vi "State_ExecCMD.vi"(6 "Callback":T1, 8 "error in (no error)":errorcluster, 9 "Parameter":variant, 10 "Command":string, 11 "MB Slave Simulator Base in":refnum<class "MB Slave Simulator Base.lvclass">) -> (0 "error out":errorcluster, 1 "Suppress Debug?":bool, 2 "Debug Message":string, 3 "MB Slave Simulator Base out":refnum<class "MB Slave Simulator Base.lvclass">)   [LabVIEW 2021, in "MB Slave Simulator Base.lvclass"]
uses:
  MB Slave Simulator Base.lvclass
  C:/Program Files (x86)/National Instruments/LabVIEW 2021/user.lib/S2 Labs/Module Framework/Modules/Modbus/Modbus Slave Base/Modbus Slave Base.lvclass
  <userlib>/S2 Labs/Module Framework/Modules/Base/Callback Typdef.ctl
  <userlib>/S2 Labs/Queued State Machine/Callback Notifier/Callback Notifier.lvclass
  <userlib>/S2 Labs/Queued State Machine/TypeDefs/CallbackNotifierRef.ctl
  TypeDefs/set_register_cmd_type.ctl
  <userlib>/S2 Labs/Module Framework/Modules/Modbus/Modbus Slave Base/Modbus Slave Base.lvclass/Modbus Slave Base.ctl
  <userlib>/S2 Labs/Queued State Machine/Callback Notifier/Callback Notifier.lvclass/Callback Notifier.ctl
  064588b5-2067-4a9b-8024-f71601e02561.vi
  780a900f-1216-485f-86c7-dbb916bac525.vi
  e8940690-14e9-4793-917b-da751b7dd203.vi
  <userlib>/S2 Labs/Module Framework/Modules/Modbus/Modbus Slave Base/Read MB Ref.vi
  <userlib>/S2 Labs/Queued State Machine/Callback Notifier/Read Callback Notifier Ref.vi
  <vilib>/Utility/error.llb/Error Cluster From Error Code.vi
  <vilib>/JDP Science/JSONtext/Variant to JSON Text.vi
  <userlib>/S2 Labs/Modbus Toolkit/Slave/S2L Modbus Slave.lvclass
  <vilib>/JDP Science/JSONtext/LVClass Serializer/JSONtext LVClass Serializer.lvclass
  <userlib>/S2 Labs/Module Framework/Modules/Modbus/Modbus Slave Base/Modbus Slave Base.lvclass
  <userlib>/S2 Labs/Queued State Machine/QSM.lvclass
  <userlib>/S2 Labs/Module Framework/Modules/Base/Module.lvclass
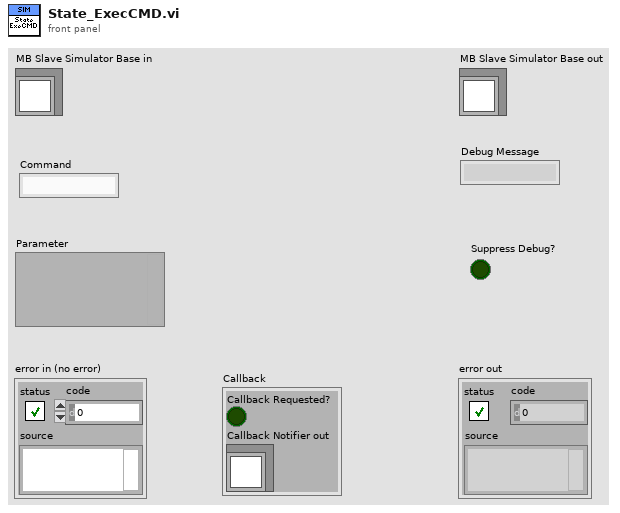
[diagram p1: front panel]
types:
  T1 = typedef "Module.lvclass/Callback Typdef.ctl" = cluster{"Callback Requested?":bool, "Callback Notifier out":T2}
  T2 = typedef "QSM.lvclass/CallbackNotifierRef.ctl" = refnum<class "Callback Notifier.lvclass">
  T3 = typedef "MB Slave Simulator Base.lvclass/set_register_cmd_type.ctl" = cluster{"Label":string, "Value":dbl}
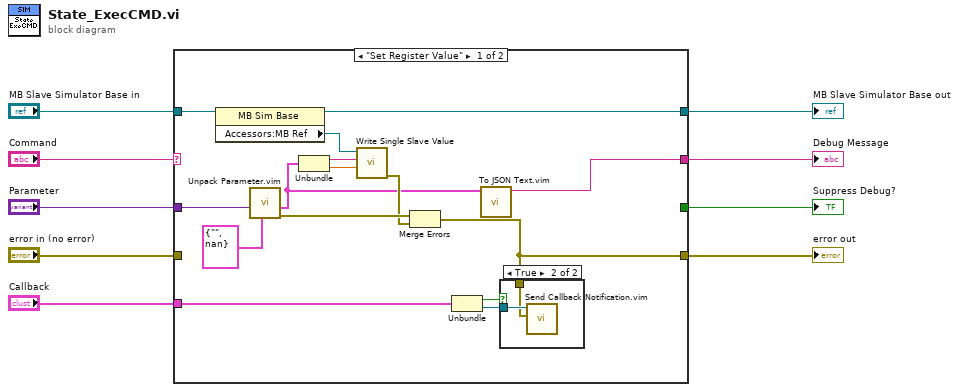
[diagram p0: block diagram]
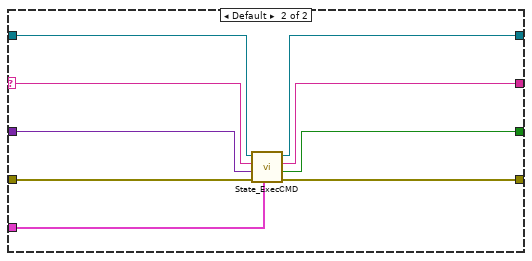
[diagram p3: hidden frame]
diagram:
  n1 = case shown="\"Set Register Value\"" "Command" {
    selector: "Command" -> [_ w28]
    tunnel: [w12 w35] -> w9
    tunnel: [_ w34] -> w8
    tunnel: [w10 w33] -> w7
    tunnel: [w23 w32] -> w6
    tunnel: "Callback" -> [w21 w31]
    tunnel: "error in (no error)" -> [_ w30]
    tunnel: "Parameter" -> [w18 w29]
    tunnel: "MB Slave Simulator Base in" -> [w24 w27]
    frame "Set Register Value" {
      n2 = property class="MB Sim Base"(reference=w24) -> (reference out=w23:refnum<class "MB Slave Simulator Base.lvclass">, "Accessors:MB Ref"=w22:refnum<class "S2L Modbus Slave.lvclass">)  [unwired: 1 in, 1 out]
      n3 = call "Unpack Parameter.vim"("Parameter type (string)"=T3 {"Label"="", "Value"=nan} ("Set Register CMD"), "Parameter Variant"=w18) -> ("error out"=w14:errorcluster, "Parameter"=w11:T3)  [unwired: 8 in]
      n4 = Unbundle(w11) -> ("Label"=w16:string, "Value"=w15:dbl)
      n5 = call-dynamic "Write Single Slave Value.vi"("Value"=w15, "Label"=w16, "S2L Modbus Slave in"=w22) -> ("error out"=w13:errorcluster)  [unwired: 7 in, 1 out]
      n6 = Merge Errors(w14, w13) -> (w12:errorcluster)
      n7 = Unbundle(w21) -> ("Callback Requested?"=w20:bool, "Callback Notifier out"=w19:T2)
      n8 = call "To JSON Text.vim"("Anything"=w11) -> ("<JSON>"=w10:string)  [unwired: 9 in, 1 out]
      n9 = case shown="True" w20 {
        tunnel: w19 -> [_ w26]
        tunnel: w12 -> [_ w25]
        frame False {
        }
        frame True {
          n10 = call "Send Callback Notification.vim"("notification (string)"=w25, "Callback Notifier in"=w26) -> ()  [unwired: 8 in, 2 out]
        }
      }
    }
    frame Default {
      n11 = call-parent "State_ExecCMD.vi"("Callback"=w31, "error in (no error)"=w30, "Parameter"=w29, "Command"=w28, "Modbus Slave Base in"=w27) -> ("error out"=w35:errorcluster, "Suppress Debug?"=w34:bool, "Debug Message"=w33:string, "Modbus Slave Base out"=w32:refnum<class "MB Slave Simulator Base.lvclass">)  [unwired: 3 in]
    }
  }
  "error out" <- w9
  "MB Slave Simulator Base out" <- w6
  "Debug Message" <- w7
  "Suppress Debug?" <- w8
